vi "MainVI.vi"() -> ()   [LabVIEW 2020]
panel:
  in  "RE":bool
  in  "Down R":bool
  in  "R-L":bool
  in  "Up":bool
  in  "Hold":bool
  in  "Down":bool
  out "Boolean":bool
  out "Boolean 2":bool
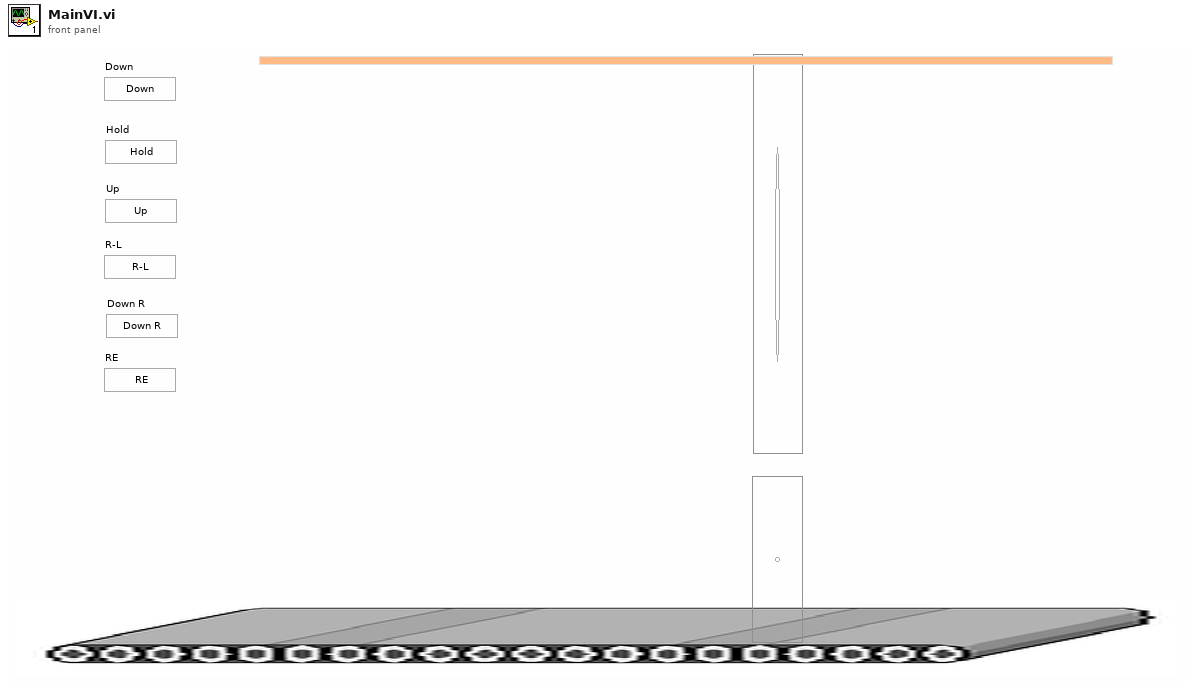
[diagram p1: front panel]
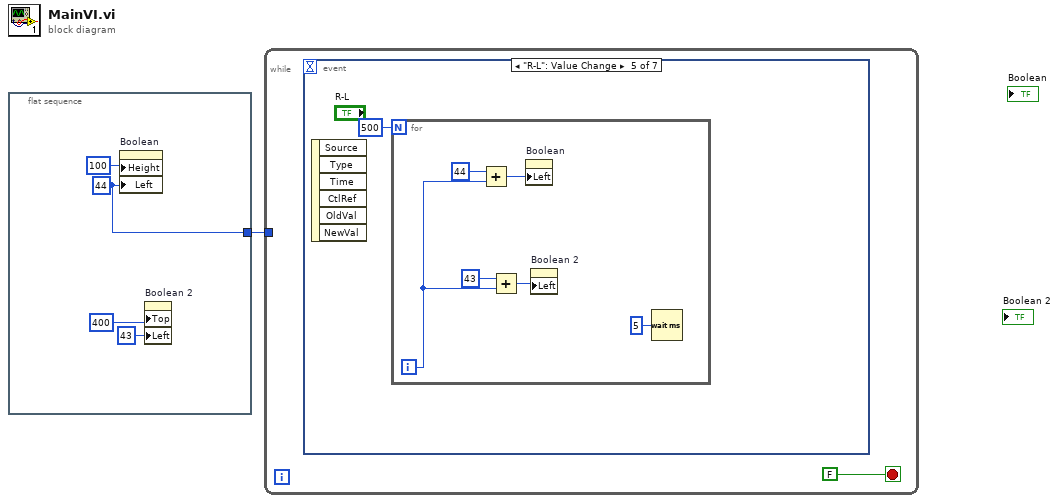
[diagram p0: block diagram]
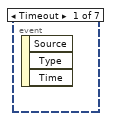
[diagram p2: hidden frame]
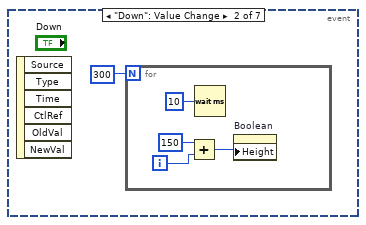
[diagram p3: hidden frame]
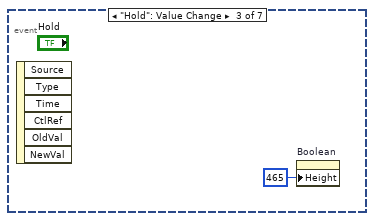
[diagram p4: hidden frame]
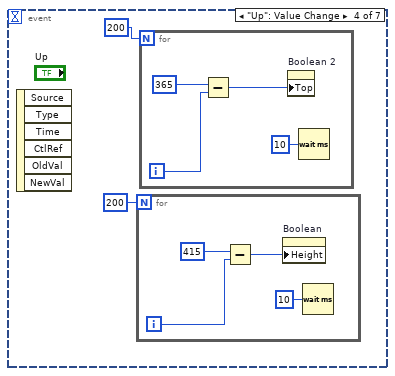
[diagram p5: hidden frame]
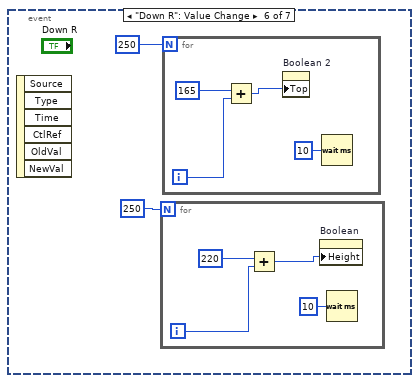
[diagram p6: hidden frame]
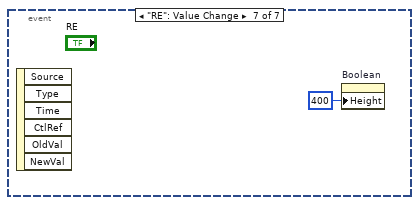
[diagram p7: hidden frame]
diagram:
  n1 = flat-sequence {
    tunnel: [w2] -> w1
    frame #0 {
      w2 = 44 ("Position:Left")
      n2 = property on="Boolean" class="Bool (strict)"("Height"=u32 100 ("Button Size:Height"), "Left"=w2) -> ()  [unwired: 2 in, 2 out]
      n3 = property on="Boolean 2" class="Bool (strict)"("Top"=400 ("Position:Top"), "Left"=43 ("Position:Left")) -> ()  [unwired: 2 in, 2 out]
    }
  }
  n4 = while {
    tunnel: w1 -> [_]
    stop <- FALSE stop-if-true
    n5 = event shown="[4] \"R-L\": Value Change" {
      selector: _ -> [_ _ _ _ _ _ _]
      dyn-events: _ -> [_ _ _ _ _ _ _]
      timeout: _ -> [_ _ _ _ _ _ _]
      event Timeout {
        n6 = event-data() -> ()  [unwired: 1 in, 3 out]
      }
      event "Down": Value Change {
        n7 = event-data() -> ()  [unwired: 1 in, 6 out]
        n8 = for {
          N: 300 -> [_]
          i -> [w9]
          n9 = Add(x=150, y=w9) -> (x+y=w8:i32)
          n10 = Wait (ms)(milliseconds to wait=u32 10) -> ()  [unwired: 1 out]
          n11 = property on="Boolean" class="Bool (strict)"("Height"=w8) -> ()  [unwired: 2 in, 2 out]
        }
      }
      event "Hold": Value Change {
        n12 = event-data() -> ()  [unwired: 1 in, 6 out]
        n13 = property on="Boolean" class="Bool (strict)"("Height"=u32 465 ("Button Size:Height")) -> ()  [unwired: 2 in, 2 out]
      }
      event "Up": Value Change {
        n14 = event-data() -> ()  [unwired: 1 in, 6 out]
        n15 = for {
          N: 200 -> [_]
          i -> [w17]
          n16 = Subtract(x=415, y=w17) -> (x-y=w15:i32)
          n17 = property on="Boolean" class="Bool (strict)"("Height"=w15) -> ()  [unwired: 2 in, 2 out]
          n18 = Wait (ms)(milliseconds to wait=u32 10) -> ()  [unwired: 1 out]
        }
        n19 = for {
          N: 200 -> [_]
          i -> [w21]
          n20 = Subtract(x=365, y=w21) -> (x-y=w19:i32)
          n21 = property on="Boolean 2" class="Bool (strict)"("Top"=w19) -> ()  [unwired: 2 in, 2 out]
          n22 = Wait (ms)(milliseconds to wait=u32 10) -> ()  [unwired: 1 out]
        }
      }
      event "R-L": Value Change {
        n23 = event-data() -> ()  [unwired: 1 in, 6 out]
        n24 = for {
          N: 500 -> [_]
          i -> [w27]
          n25 = Add(x=44, y=w27) -> (x+y=w29:i32)
          n26 = Add(x=43, y=w27) -> (x+y=w28:i32)
          n27 = property on="Boolean" class="Bool (strict)"("Left"=w29) -> ()  [unwired: 2 in, 2 out]
          n28 = property on="Boolean 2" class="Bool (strict)"("Left"=w28) -> ()  [unwired: 2 in, 2 out]
          n29 = Wait (ms)(milliseconds to wait=u32 5) -> ()  [unwired: 1 out]
        }
      }
      event "Down R": Value Change {
        n30 = event-data() -> ()  [unwired: 1 in, 6 out]
        n31 = for {
          N: 250 -> [_]
          i -> [w34]
          n32 = Add(x=220, y=w34) -> (x+y=w32:i32)
          n33 = property on="Boolean" class="Bool (strict)"("Height"=w32) -> ()  [unwired: 2 in, 2 out]
          n34 = Wait (ms)(milliseconds to wait=u32 10) -> ()  [unwired: 1 out]
        }
        n35 = for {
          N: 250 -> [_]
          i -> [w38]
          n36 = Add(x=165, y=w38) -> (x+y=w36:i32)
          n37 = property on="Boolean 2" class="Bool (strict)"("Top"=w36) -> ()  [unwired: 2 in, 2 out]
          n38 = Wait (ms)(milliseconds to wait=u32 10) -> ()  [unwired: 1 out]
        }
      }
      event "RE": Value Change {
        n39 = event-data() -> ()  [unwired: 1 in, 6 out]
        n40 = property on="Boolean" class="Bool (strict)"("Height"=u32 400 ("Button Size:Height")) -> ()  [unwired: 2 in, 2 out]
      }
    }
  }
